vi "DetectCollisionSmoother.vi"(0 "Goal":dbl[](array[numeric]), 4 "Initial State":dbl[](array[numeric]), 6 "enemy_robots":T1[](array[typedef]), 7 "Robot in":T1, 8 "SegmentPointB":dbl[](array[numeric]), 9 "SegmentPointA":dbl[](array[numeric])) -> (3 "Is there colision?":bool)   [LabVIEW 2017]
uses:
  Core/AI Robot.ctl
  Intel/Functions Enum.ctl
  Intel/AttackerStates.ctl
  PathDests.ctl
  PathDest.ctl
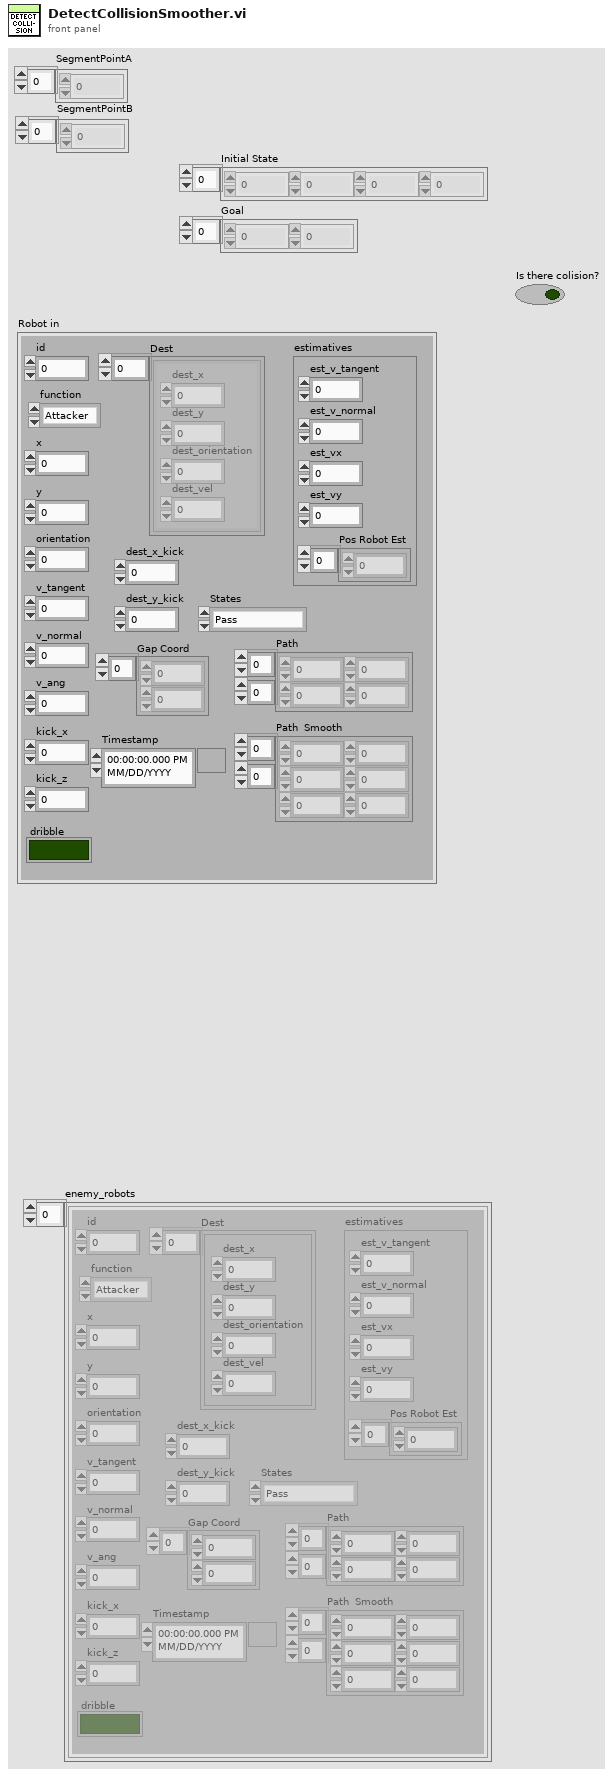
[diagram p1: front panel]
types:
  T1 = typedef "AI Robot.ctl" = cluster{"id":u32, "function":T2, "x":dbl, "y":dbl, "orientation":dbl, "v_tangent":dbl, "v_normal":dbl, "v_ang":dbl, "kick_x":dbl, "kick_z":dbl, "dribble":bool, "Timestamp":timestamp, "estimatives":cluster{"est_v_tangent":dbl, "est_v_normal":dbl, "est_vx":dbl, "est_vy":dbl, "Pos Robot Est":dbl[]}, "dest_x_kick":dbl, "dest_y_kick":dbl, "Gap Coord":dbl[], "States":T3, "Path ":dbl[][], "Path  Smooth":dbl[][], "Dest":T4}
  T2 = typedef "Functions Enum.ctl" = enum16{"Attacker", "Goalie", "Defender", "Striker", "Goto 0", "Dummy", "Kicker", "ZigZag"}
  T3 = typedef "AttackerStates.ctl" = enum16{"Pass", "GoToTangent", "BallGetting", "GoToKick", ""}
  T4 = typedef "PathDests.ctl" = T5[]
  T5 = typedef "PathDest.ctl" = cluster{"dest_x":dbl, "dest_y":dbl, "dest_orientation":dbl, "dest_vel":dbl}
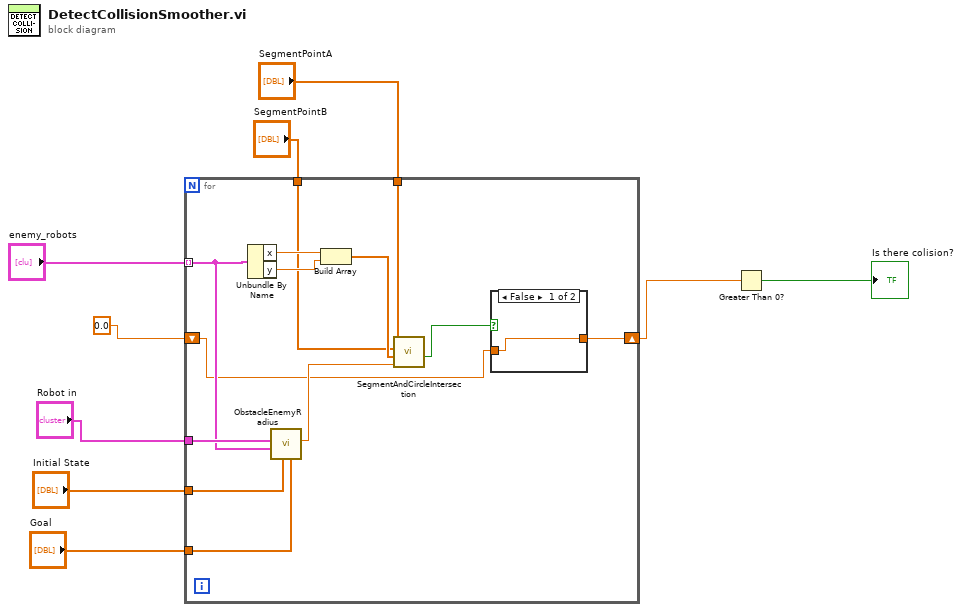
[diagram p0: block diagram]
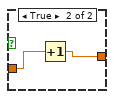
[diagram p2: hidden frame]
diagram:
  n1 = for {
    tunnel: "enemy_robots" -> [w16] mode=indexing
    tunnel: "Initial State" -> [w19]
    tunnel: "Goal" -> [w18]
    tunnel: "Robot in" -> [w17]
    tunnel: "SegmentPointA" -> [w14]
    tunnel: "SegmentPointB" -> [w13]
    shift-right: [w10] -> w1
    shift-left: 0.0 -> [w11]
    n2 = Unbundle By Name(w16) -> ("x"=w22:dbl, "y"=w21:dbl)
    n3 = call "ObstacleEnemyRadius.vi"("Goal"=w18, "Initial State"=w19, "Robot enemy"=w16, "Robot in"=w17) -> ("obstacle enemy radius"=w15:dbl)  [unwired: 7 in]
    n4 = Build Array(w22, w21) -> (w20:dbl[])
    n5 = call "SegmentAndCircleIntersection.vi"("CircleRadius"=w15, "CircleCenter"=w20, "SegmentPointB"=w13, "SegmentPointA"=w14) -> ("DoTheyIntersect?"=w12:bool)  [unwired: 7 in]
    n6 = case shown="False" w12 {
      tunnel: w11 -> [w23 w25]
      tunnel: [w23 w24] -> w10
      frame False {
      }
      frame True {
        n7 = Increment(x=w25) -> (x+1=w24:dbl)
      }
    }
  }
  n8 = Greater Than 0?(x=w1) -> (x > 0?=→"Is there colision?":bool)
